vi "GetCountOverflow.vi"() -> (2 "overflow":bool, 3 "count":i32)   [LabVIEW 2014]
uses:
  USBAnalyzerEllisysDll.dll
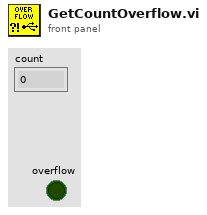
[diagram p1: front panel]
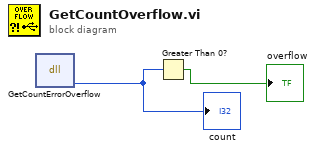
[diagram p0: block diagram]
diagram:
  n1 = dll-call lib="PTH2Wabs CUsersMichał\tDocumentsEllisysAnalyzerLabVIEWUSBAnalyzerEllisysDll.dll" fn="GetCountErrorOverflow"() -> ("count"=w2:i32)  [unwired: 5 in, 2 out]
  "count" <- w2
  n2 = Greater Than 0?(x=w2) -> (x > 0?=→"overflow":bool)
